vi "Read Nitro.vi"(11 "FPGA API in":refnum<class "FPGA API.lvclass">) -> (2 "Nitro":bool, 3 "FPGA API out":refnum<class "FPGA API.lvclass">)   [LabVIEW 2019, in "FPGA API.lvclass"]
uses:
  FPGA API.lvclass
  FPGA API.lvclass/FPGA API.ctl
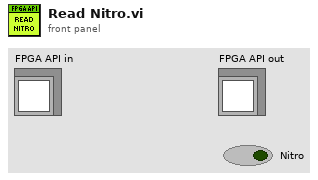
[diagram p1: front panel]
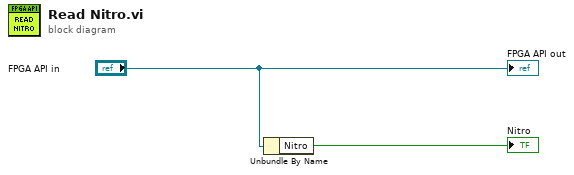
[diagram p0: block diagram]
diagram:
  n1 = Unbundle By Name("FPGA API in") -> ("Nitro"=→"Nitro":bool)
  "FPGA API out" <- "FPGA API in"
